vi "MultiOpto_1.1_Begin.vi"() -> (0 "NI Scope Status":bool, 1 "Stepper Motor Status":bool, 2 "Ophir 2 Status":bool, 3 "Ophir 1 Status":bool, 4 "Текущий Образец №":string, 5 "NI DMM 2 option return":enum32{"Ampermeter button", "Ohmmeter button"}(ring), 6 "NI DMM 3 option return":enum32{"Ampermeter button", "Ohmmeter button"}(ring), 7 "NI DMM 1 option return":enum32{"Ampermeter button", "Ohmmeter button"}(ring), 9 "NI DMM 3 Status":bool, 10 "NI DMM 2 Status":bool, 11 "NI DMM 1 Status":bool)   [LabVIEW 2018]
panel:
  in  "OK Button":bool
  in  "Stepper Motor":bool
  in  "NI DMM 3 option":enum32{"Ampermeter button", "Ohmmeter button"}(radio)
  in  "NI DMM 3":bool
  in  "NI DMM 2 option":enum32{"Ampermeter button", "Ohmmeter button"}(radio)
  in  "NI DMM 1 option":enum32{"Ampermeter button", "Ohmmeter button"}(radio)
  in  "Ophir 2":bool
  in  "NI DMM 2":bool
  out "Boolean 4":bool
  out "Boolean 3":bool
  in  "Ophir 1":bool
  in  "NI DMM 1":bool
  in  "NI Scope":bool
  in  "Образец №":string
  out "Boolean":bool
  out "Boolean 2":bool
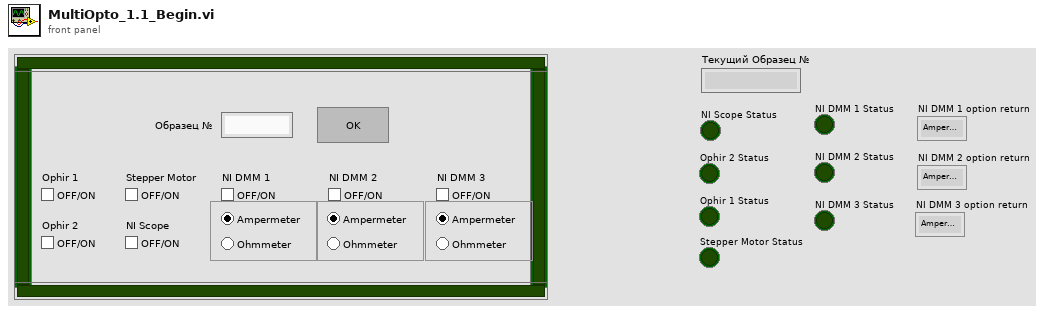
[diagram p1: front panel]
types:
  T1 = enum8{"Enabled", "Disabled", "Disabled and Grayed Out"}
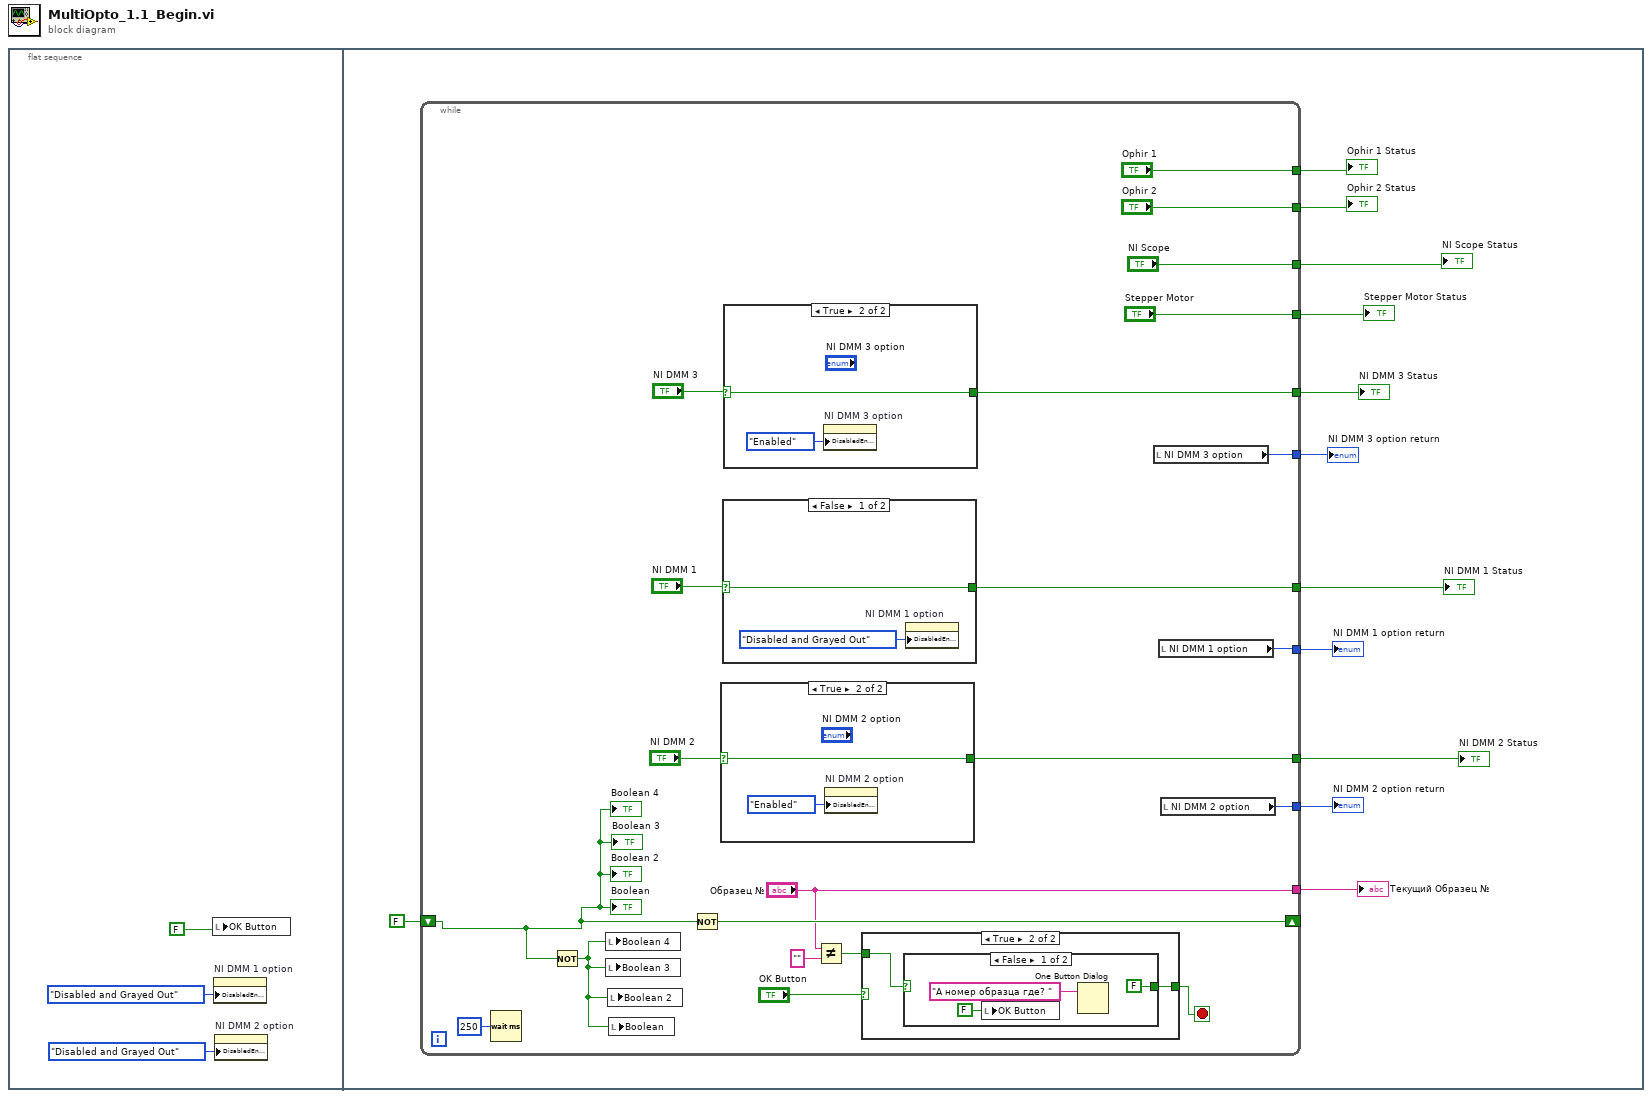
[diagram p0: block diagram]
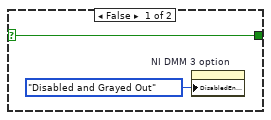
[diagram p4: hidden frame]
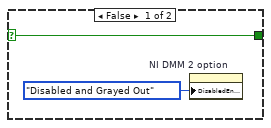
[diagram p5: hidden frame]
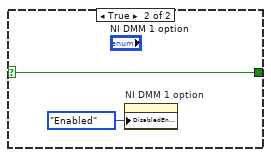
[diagram p6: hidden frame]
diagram:
  n1 = flat-sequence {
    frame #0 {
      n2 = local write "OK Button"(FALSE ("Ввел!")) -> ()
      n3 = property on="NI DMM 1 option" class="RadioBtnsControl (strict)"("DisabledEnum"=T1."Disabled and Grayed Out" ("Disabled")) -> ()  [unwired: 2 in, 2 out]
      n4 = property on="NI DMM 2 option" class="RadioBtnsControl (strict)"("DisabledEnum"=T1."Disabled and Grayed Out" ("Disabled")) -> ()  [unwired: 2 in, 2 out]
    }
    frame #1 {
      n5 = while {
        tunnel: ["Образец №"] -> w15
        shift-right: [w36] -> _
        shift-left: FALSE -> [w35]
        tunnel: ["NI Scope"] -> w13
        tunnel: [w28] -> w12
        tunnel: ["Ophir 1"] -> w11
        tunnel: [w27] -> w10
        tunnel: ["Ophir 2"] -> w9
        tunnel: [w26] -> w8
        tunnel: [w25] -> w7
        tunnel: [w23] -> w6
        tunnel: [w22] -> w5
        tunnel: ["Stepper Motor"] -> w4
        stop <- w18 stop-if-true
        n6 = Wait (ms)(milliseconds to wait=u32 250) -> ()  [unwired: 1 out]
        n7 = Not(x=w35) -> (.not. x?=w34:bool)
        n8 = local write "Boolean 4"(w34) -> ()
        n9 = local write "Boolean 3"(w34) -> ()
        n10 = local write "Boolean 2"(w34) -> ()
        n11 = local write "Boolean"(w34) -> ()
        n12 = Not(x=w35) -> (.not. x?=w36:bool)
        n13 = case shown="True" "NI DMM 2" {
          selector: "NI DMM 2" -> [w49 w52]
          tunnel: [w49 w52] -> w27
          frame False {
            n14 = property on="NI DMM 2 option" class="RadioBtnsControl (strict)"("DisabledEnum"=T1."Disabled and Grayed Out" ("Disabled")) -> ()  [unwired: 2 in, 2 out]
          }
          frame True {
            n15 = property on="NI DMM 2 option" class="RadioBtnsControl (strict)"("DisabledEnum"=T1."Enabled" ("Disabled")) -> ()  [unwired: 2 in, 2 out]
          }
        }
        n16 = case shown="False" "NI DMM 1" {
          selector: "NI DMM 1" -> [w53 w56]
          tunnel: [w53 w56] -> w28
          frame False {
            n17 = property on="NI DMM 1 option" class="RadioBtnsControl (strict)"("DisabledEnum"=T1."Disabled and Grayed Out" ("Disabled")) -> ()  [unwired: 2 in, 2 out]
          }
          frame True {
            n18 = property on="NI DMM 1 option" class="RadioBtnsControl (strict)"("DisabledEnum"=T1."Enabled" ("Disabled")) -> ()  [unwired: 2 in, 2 out]
          }
        }
        n19 = case shown="True" "NI DMM 3" {
          selector: "NI DMM 3" -> [w45 w48]
          tunnel: [w45 w48] -> w23
          frame False {
            n20 = property on="NI DMM 3 option" class="RadioBtnsControl (strict)"("DisabledEnum"=T1."Disabled and Grayed Out" ("Disabled")) -> ()  [unwired: 2 in, 2 out]
          }
          frame True {
            n21 = property on="NI DMM 3 option" class="RadioBtnsControl (strict)"("DisabledEnum"=T1."Enabled" ("Disabled")) -> ()  [unwired: 2 in, 2 out]
          }
        }
        n22 = Not Equal?(x="Образец №", y="") -> (x != y?=w19:bool)
        n23 = case shown="True" "OK Button" {
          selector: "OK Button" -> [w38 _]
          tunnel: w19 -> [_ w40]
          tunnel: [w38 w39] -> w18
          frame False {
          }
          frame True {
            n24 = case shown="False" w40 {
              selector: w40 -> [_ w44]
              tunnel: [FALSE w44] -> w39
              frame False {
                n25 = local write "OK Button"(FALSE ("OK Button")) -> ()
                n26 = One Button Dialog(message="А номер образца где? ") -> ()  [unwired: 1 in, 1 out]
              }
              frame True {
              }
            }
          }
        }
        n27 = local read "NI DMM 3 option"() -> (w22:enum32{"Ampermeter button", "Ohmmeter button"})
        n28 = local read "NI DMM 1 option"() -> (w26:enum32{"Ampermeter button", "Ohmmeter button"})
        n29 = local read "NI DMM 2 option"() -> (w25:enum32{"Ampermeter button", "Ohmmeter button"})
        "Boolean" <- w35
        "Boolean 2" <- w35
        "Boolean 3" <- w35
        "Boolean 4" <- w35
      }
      "Текущий Образец №" <- w15
      "NI Scope Status" <- w13
      "NI DMM 1 Status" <- w12
      "Ophir 1 Status" <- w11
      "NI DMM 2 Status" <- w10
      "Ophir 2 Status" <- w9
      "NI DMM 2 option return" <- w7
      "NI DMM 1 option return" <- w8
      "NI DMM 3 Status" <- w6
      "NI DMM 3 option return" <- w5
      "Stepper Motor Status" <- w4
    }
  }
